vi "MessageBox.vi"(5 "message":string, 6 "Default Button":T1(ring), 7 "Icon Type":T2(ring), 8 "Button Types":T3(ring), 9 "caption":string) -> (2 "Output Value":i32)   [LabVIEW 2012]
uses:
  user32.dll
  bin/LtMessageBox.dll
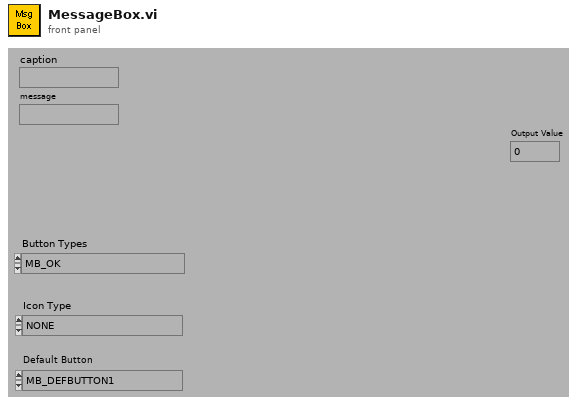
[diagram p1: front panel]
types:
  T1 = enum16{"MB_DEFBUTTON1", "MB_DEFBUTTON2", "MB_DEFBUTTON3"}
  T2 = enum16{"NONE", "MB_ICONHAND", "MB_ICONQUESTION", "MB_ICONEXCLAMATION", "MB_ICONINFORMATION"}
  T3 = enum16{"MB_OK", "MB_OKCANCEL", "MB_ABORTRETRYIGNORE", "MB_YESNOCANCEL", "MB_YESNO", "MB_RETRYCANCEL"}
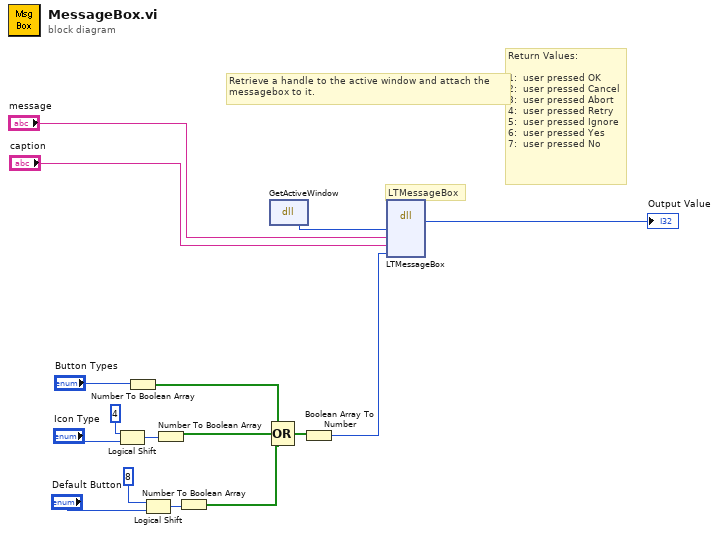
[diagram p0: block diagram]
diagram:
  # "Retrieve a handle to the active window and attach the\nmessagebox to it."
  # "Return Values:\n\n1:  user pressed OK\n2:  user pressed Cancel\n3:  user pressed Abort\n4:  user pressed Retry\n5:  user pressed Ignore\n6:  user pressed Yes\n7:  user pressed No"
  # "LTMessageBox"
  n1 = Logical Shift(y=4, x="Icon Type") -> (x << y=w13:u32)
  n2 = Number To Boolean Array(number="Button Types") -> (Boolean array=w10:bool[])
  n3 = Logical Shift(y=8, x="Default Button") -> (x << y=w11:u32)
  n4 = Number To Boolean Array(number=w13) -> (Boolean array=w9:bool[])
  n5 = Number To Boolean Array(number=w11) -> (Boolean array=w8:bool[])
  n6 = dll-call lib="user32.dll" fn="GetActiveWindow"() -> (w1:u32)  [unwired: 3 in, 2 out]
  n7 = Compound Arithmetic op=OR(w10, w9, w8) -> (w7:bool[])
  n8 = Boolean Array To Number(Boolean array=w7) -> (number=w6:u32)
  n9 = dll-call lib="C:/_src/OVA5000_DSP_falcon/Software/LabVIEW/OVA/SDK/OVA_5000_SDK_v5.14.3/bin/LtMessageBox.dll" fn="LTMessageBox"("HWND"=w1, "message"="message", "caption"="caption", "type"=w6) -> ("return type"=→"Output Value":i32)  [unwired: 7 in, 2 out]
